vi "tb_LUT.vi"(7 "FFT Size":T1=enum."8192", 9 "Reset?":bool) -> ()   [LabVIEW 2011]
doc: "This VI generates twiddle factors for sine and cosine generation\n\n<b> Latency = 16 Ticks </b>"
uses:
  <userlib>/FPGA Library/Code Development/Signal Processing/FFT Block/FFT/FFT Size.ctl
  <vilib>/rvi/IPIntegrationNode/IPINode_Utilities/niFpgaIPINodeSimCore.vi
  <vilib>/rvi/FXPMathLib/FxpInterpret/XNode/nifxpmath_Interpret.xnode
  <vilib>/rvi/XilinxIP/XIPIN_XNode/niFpgaXIPIN.xnode
  <userlib>/FPGA Library/Code Development/Signal Processing/FFT Block/Twiddle Factor/LUT/SinCosLUT_4AF2FDD64E94328E5B0A30B3AC6E6500.dll
  <vilib>/rvi/IPIntegrationNode/IPINode_Xnode/niFpgaIPINode.xnode
panel:
  out "cos(x)":dbl[](array[numeric])
  out "Cosine":fxp<+/-,18,2>[](array[numeric])
  out "Sine":fxp<+/-,18,2>[](array[numeric])
  out "sin(x)":dbl[](array[numeric])
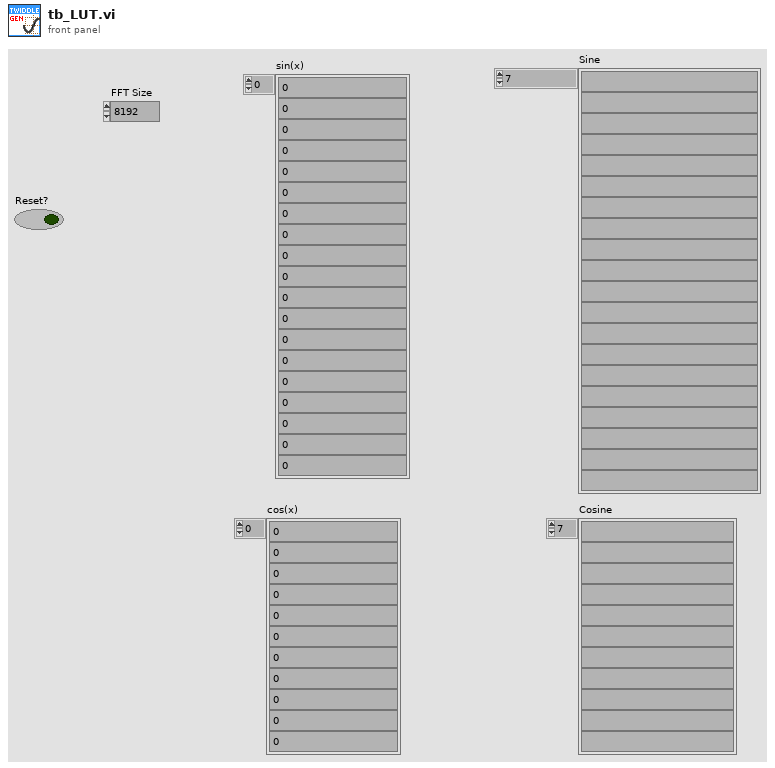
[diagram p1: front panel]
types:
  T1 = typedef "FFT Size.ctl" = enum16{"512", "1024", "2048", "4096", "8192", "16384", "32768"}
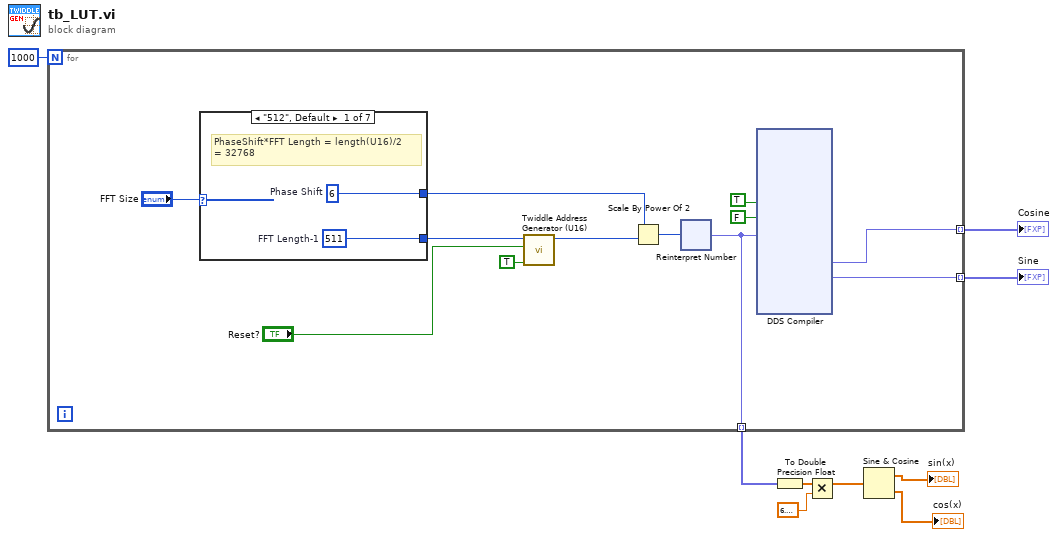
[diagram p0: block diagram]
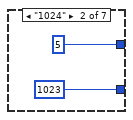
[diagram p2: hidden frame]
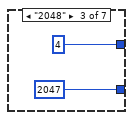
[diagram p3: hidden frame]
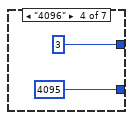
[diagram p4: hidden frame]
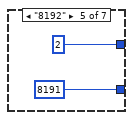
[diagram p5: hidden frame]
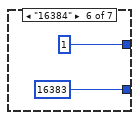
[diagram p6: hidden frame]
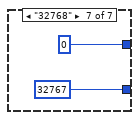
[diagram p7: hidden frame]
diagram:
  n1 = for {
    N: 1000 -> [_]
    tunnel: [w12] -> w9 mode=indexing
    tunnel: [w11] -> w7 mode=indexing
    tunnel: [w10] -> w5 mode=indexing
    n2 = case shown="\"512\", Default" "FFT Size" {
      tunnel: [w90 u8 5 ("n") u8 4 ("n") u8 3 ("n") u8 2 ("n") u8 1 ("n") u8 0 ("n")] -> w20
      tunnel: [w89 u16 1023 u16 2047 u16 4095 u16 8191 u16 16383 u16 32767] -> w19
      frame "512", Default {
        w89 = u16 511  # FFT Length-1
        w90 = u8 6  # Phase Shift
        # "PhaseShift*FFT Length = length(U16)/2\n= 32768"
      }
      frame "1024" {
      }
      frame "2048" {
      }
      frame "4096" {
      }
      frame "8192" {
      }
      frame "16384" {
      }
      frame "32768" {
      }
    }
    n3 = call <userlib>:"Twiddle Address Generator (U16).vi"("INC?"=TRUE, "Reset?"="Reset?", "rollover"=w19) -> ("count"=w17:u16)  [unwired: 8 in]
    n4 = Scale By Power Of 2(n=w20, x=w17) -> (x*2^n=w15:u16)
    n5 = xnode "Reinterpret Number"("x"=w15) -> ("y"=w12:fxp<+,16,0>)
    n6 = xnode ("DDS Compiler")("ce"=TRUE, "sclr"=FALSE, "phase_in"=w12) -> ("cosine"=w10:fxp<+/-,18,2>, "sine"=w11:fxp<+/-,18,2>)  [unwired: 3 out]
  }
  "Sine" <- w7
  "Cosine" <- w5
  n7 = To Double Precision Float(number=w9) -> (double precision float=w8:dbl[])
  n8 = Multiply(x=w8, y=6.283185307179586) -> (x*y=w2:dbl[])
  n9 = Sine & Cosine(0:w2) -> (1:→"sin(x)":dbl[], 2:→"cos(x)":dbl[])
